vi "std get cycle seq results.vi"(8 "error in":errorcluster) -> (3 "cycle results cluster out":T1, 11 "cycle results cluster IN":T1)   [LabVIEW 2016]
doc: "Takes a sample type and sorts by sequence"
uses:
  controls/cycle results control.ctl
  <vilib>/Analysis/baseanly.llb/Mean (DBL).vi
  <vilib>/Analysis/NI_AALBase.lvlib
panel:
  out "error out":errorcluster
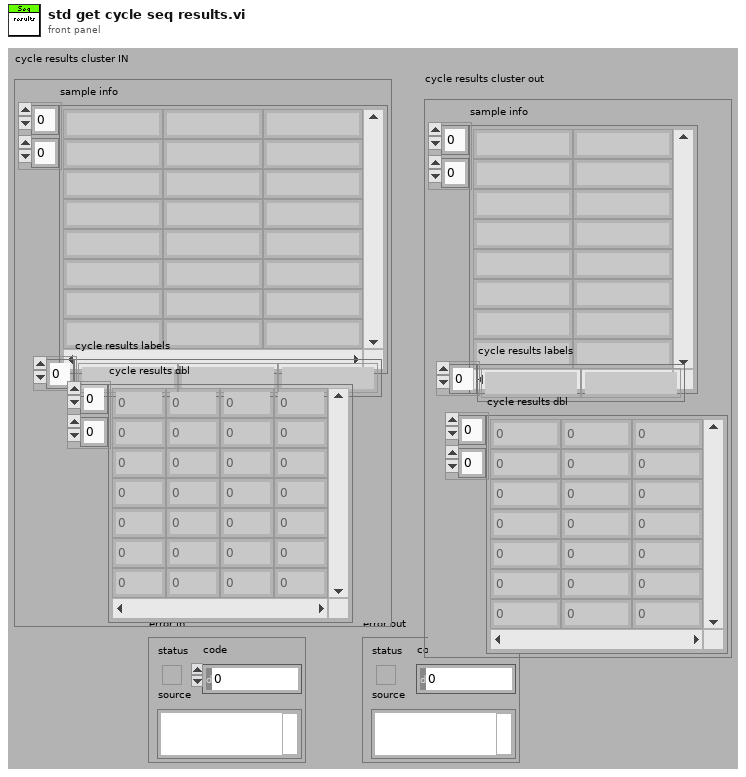
[diagram p1: front panel]
types:
  T1 = typedef "cycle results control.ctl" = cluster{"sample info":string[][], "cycle results labels":string[], "cycle results dbl":dbl[][]}
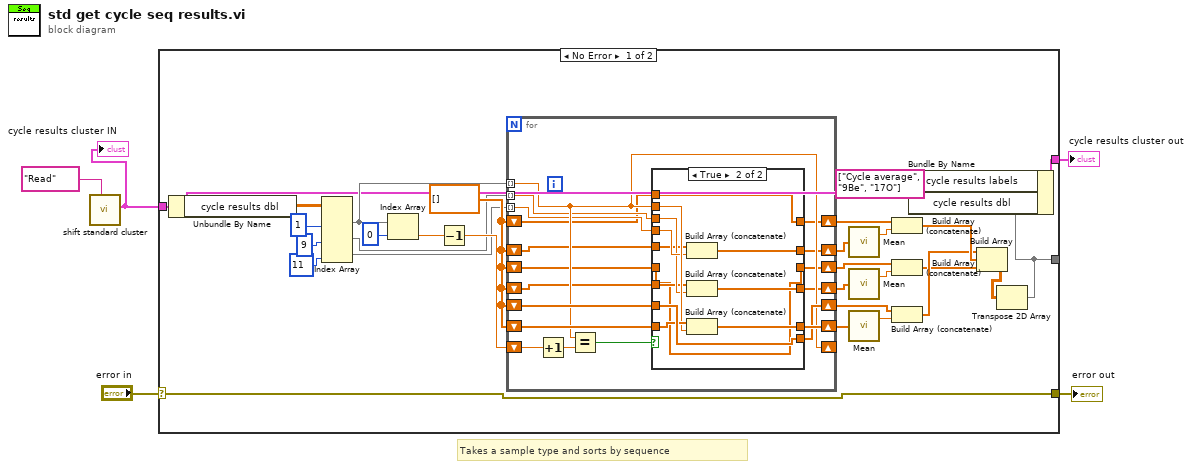
[diagram p0: block diagram]
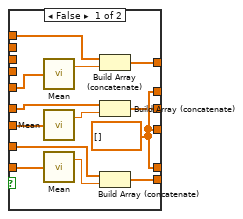
[diagram p2: hidden frame]
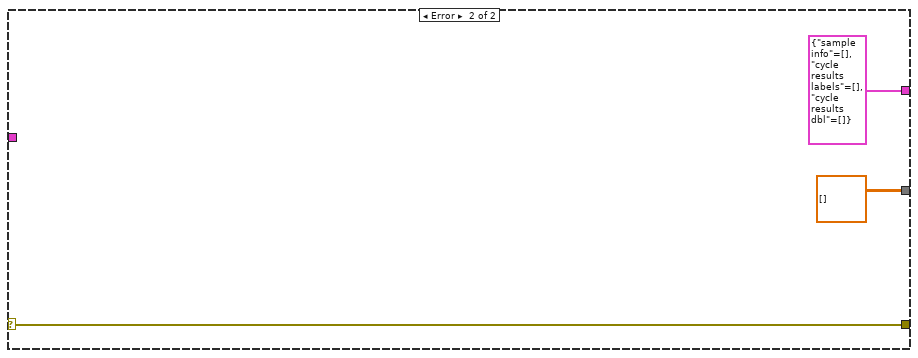
[diagram p3: hidden frame]
diagram:
  # "Takes a sample type and sorts by sequence"
  n1 = call "shift standard cluster.vi"("read write shift"="Read") -> ("cycle results cluster out"=w1:T1)  [unwired: 9 in, 1 out]
  "cycle results cluster IN" <- w1
  n2 = case shown="No Error" "error in" {
    selector: "error in" -> [w11 w79]
    tunnel: w1 -> [w10 _]
    tunnel: [w6 dbl[][] []] -> _
    tunnel: [w8 T1 {"sample info"=[], "cycle results labels"=[], "cycle results dbl"=[]} ("cycle results cluster IN")] -> w3
    tunnel: [w11 w79] -> w4
    frame No Error {
      w24 = dbl[] []
      n3 = Unbundle By Name(w10) -> ("cycle results dbl"=w21:dbl[][])
      n4 = Index Array(array=w21, index (col) #1=1 ("disabled index (col)"), index (col) #2=9 ("index (col)"), index (col) #3=11 ("index (col)")) -> (element #1=w17:dbl[], element #2=w16:dbl[], element #3=w15:dbl[])  [unwired: 3 in]
      n5 = Index Array(array=w17, index=0) -> (element=w25:dbl)
      n6 = Decrement(x=w25) -> (x-1=w23:dbl)
      n7 = for {
        tunnel: w17 -> [w46] mode=indexing
        shift-right: [w50] -> w27
        shift-left: w24 -> [w49]
        shift-right: [w48] -> w34
        shift-left: w24 -> [w47]
        shift-right: [w46] -> _
        shift-left: w23 -> [w52]
        tunnel: w15 -> [w45] mode=indexing
        tunnel: w16 -> [w44] mode=indexing
        shift-right: [w43] -> w26
        shift-left: w24 -> [w40]
        shift-right: [w42] -> w28
        shift-left: w24 -> [w41]
        shift-right: [w39] -> w29
        shift-left: w24 -> [w37]
        shift-right: [w38] -> w32
        shift-left: w24 -> [w36]
        n8 = Increment(x=w52) -> (x+1=w35:dbl)
        n9 = Equal?(x=w46, y=w35) -> (x = y?=w51:bool)
        n10 = case shown="True" w51 {
          tunnel: w46 -> [_ w74]
          tunnel: [w57 w77] -> w50
          tunnel: w49 -> [w65 w75]
          tunnel: [w64 w76] -> w48
          tunnel: w47 -> [w63 w76]
          tunnel: w45 -> [_ w73]
          tunnel: w44 -> [_ w72]
          tunnel: [w57 w71] -> w43
          tunnel: [w57 w70] -> w42
          tunnel: w41 -> [w59 w69]
          tunnel: w40 -> [w58 w68]
          tunnel: [w56 w67] -> w39
          tunnel: [w55 w66] -> w38
          tunnel: w37 -> [w54 w67]
          tunnel: w36 -> [w53 w66]
          frame False {
            w57 = dbl[] []
            n11 = call-poly <vilib>:"Mean.vi"("X"=w59) -> ("mean"=w60:dbl)  [unwired: 1 out]
            n12 = call-poly <vilib>:"Mean.vi"("X"=w58) -> ("mean"=w61:dbl)  [unwired: 1 out]
            n13 = call-poly <vilib>:"Mean.vi"("X"=w65) -> ("mean"=w62:dbl)  [unwired: 1 out]
            n14 = Build Array (concatenate)(w54, w60) -> (w56:dbl[])
            n15 = Build Array (concatenate)(w53, w61) -> (w55:dbl[])
            n16 = Build Array (concatenate)(w63, w62) -> (w64:dbl[])
          }
          frame True {
            n17 = Build Array (concatenate)(w69, w73) -> (w70:dbl[])
            n18 = Build Array (concatenate)(w68, w72) -> (w71:dbl[])
            n19 = Build Array (concatenate)(w75, w74) -> (w77:dbl[])
          }
        }
      }
      n20 = call-poly <vilib>:"Mean.vi"("X"=w28) -> ("mean"=w30:dbl)  [unwired: 1 out]
      n21 = call-poly <vilib>:"Mean.vi"("X"=w26) -> ("mean"=w31:dbl)  [unwired: 1 out]
      n22 = call-poly <vilib>:"Mean.vi"("X"=w27) -> ("mean"=w33:dbl)  [unwired: 1 out]
      n23 = Build Array (concatenate)(w29, w30) -> (w14:dbl[])
      n24 = Build Array (concatenate)(w32, w31) -> (w12:dbl[])
      n25 = Build Array (concatenate)(w34, w33) -> (w13:dbl[])
      n26 = Build Array(w13, w14, w12) -> (w7:dbl[][])
      n27 = Transpose 2D Array(2D array=w7) -> (transposed array=w6:dbl[][])
      n28 = Bundle By Name(cluster=w10, "cycle results labels"=string[] ["Cycle average", "9Be", "17O"], "cycle results dbl"=w6) -> (w8:T1)
    }
    frame Error {
    }
  }
  "error out" <- w4
  "cycle results cluster out" <- w3
